vi "Before Iterative Read.vi"(8 "Error In":errorcluster, 10 "Temporary File":string, 11 "SFTP":refnum<class "SFTP.lvclass">) -> (0 "Error Out":errorcluster, 2 "Local File":refnum<file>, 3 "SFTP File":refnum<class "SFTP File.lvclass">)   [LabVIEW 2018, in "Tests.lvlib" / "SFTP File.lvlib"]
uses:
  SFTP File.lvlib
  src/Toolkit/SFTP/SFTP.lvclass
  src/Toolkit/SFTP File/SFTP File.lvclass
  src/Toolkit/SFTP File/API/Typedefs/Flags.ctl
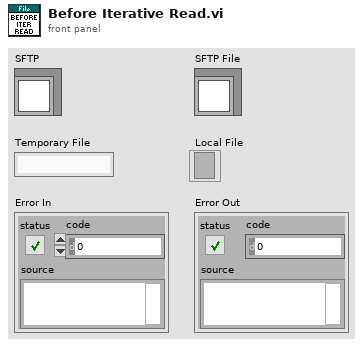
[diagram p1: front panel]
types:
  T1 = enum16{"open", "replace", "create", "open or create", "replace or create", "replace or create with confirmation"}
  T2 = typedef "Toolkit.lvlib/SFTP File.lvclass/Flags.ctl" = cluster{"Read":bool, "Write":bool, "Append":bool, "Create":bool, "Truncate":bool, "Exclude":bool}
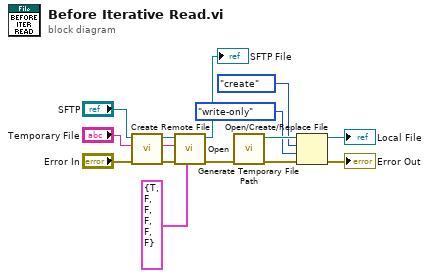
[diagram p0: block diagram]
diagram:
  n1 = call "Create Remote File.vi"("Error In"="Error In", "Remote Path In"="Temporary File", "SFTP In"="SFTP") -> ("Error Out"=w12:errorcluster, "Remote Path Out"=w11:string, "SFTP Out"=w10:refnum<class "SFTP.lvclass">)  [unwired: 6 in]
  n2 = call "Open.vi"("Flags"=T2 {"Read"=TRUE, "Write"=FALSE, "Append"=FALSE, "Create"=FALSE, "Truncate"=FALSE, "Exclude"=FALSE}, "Error In"=w12, "Remote Path"=w11, "SFTP"=w10) -> ("Error Out"=w3:errorcluster, "SFTP File"=→"SFTP File":refnum<class "SFTP File.lvclass">)  [unwired: 6 in]
  n3 = call <vilib>:"Generate Temporary File Path.vi"("error in (no error)"=w3) -> ("error out"=w7:errorcluster, "Unique Temporary File Path"=w6:path)  [unwired: 9 in]
  n4 = Open/Create/Replace File(file path (use dialog)=w6, error in=w7, operation (0:open)=T1."create", access (0:read/write)=enum16{"read/write", "read-only", "write-only"}."write-only") -> (refnum out=→"Local File":refnum<file>, error out=→"Error Out":errorcluster)  [unwired: 2 in, 1 out]
